vi "Startup.vi"(6 "DataQueues":refnum<class "DataQueues.lvclass">, 8 "error in (no error)":errorcluster, 10 "DAQ Settings*":T1, 11 "DAQ":refnum<class "DAQ.lvclass">) -> (0 "error out":errorcluster, 3 "DAQ":refnum<class "DAQ.lvclass">)   [LabVIEW 2022 SP3, in "DAQ.lvclass"]
doc: "Developed by Kevin Thompson\nkevin@thompsonengineering.net\n\nCopyright 2018-2020\nThompson Engineering, LLC"
uses:
  DAQ.lvclass
  Support/DataQueues/DataQueues.lvclass
  DataTypes/TD DAQ Settings--cluster.ctl
  DataTypes/TD DI Instrument Settings--cluster.ctl
  DataTypes/TD AI Instrument Settings--cluster.ctl
  DataTypes/TD AI InstSettings--cluster.ctl
  Process/ProcessSupport/TD SimAI Ranges--cluster.ctl
  DataTypes/TD DAQ&TDMS State Data--cluster.ctl
  DataTypes/TD DaqState--enum.ctl
  DataTypes/Dependency--cluster.ctl
  DAQ.lvclass/DAQ.ctl
  Accessors/Set DAQNodes Dict.vi
  Accessors/Set DAQData Dict.vi
  Accessors/Set DAQ&TDMS State Data.vi
  Accessors/Set DAQ Settings.vi
  Accessors/Set Dependency.vi
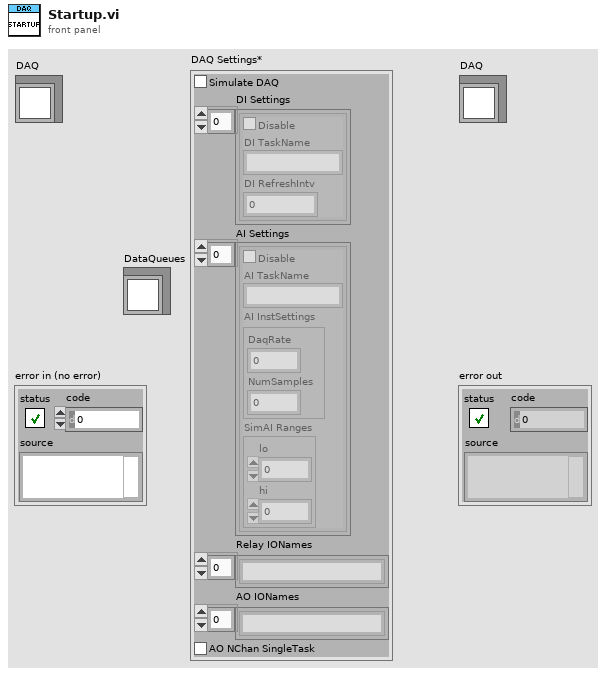
[diagram p1: front panel]
types:
  T1 = typedef "DAQ.lvclass/TD DAQ Settings--cluster.ctl" = cluster{"Simulate DAQ":bool, "DI Settings":T2[], "AI Settings":T3[], "Relay IONames":string[], "AO IONames":string[], "AO NChan SingleTask":bool}
  T2 = typedef "DAQ.lvclass/TD DI Instrument Settings--cluster.ctl" = cluster{"Disable":bool, "DI TaskName":string, "DI RefreshIntv":i32}
  T3 = typedef "DAQ.lvclass/TD AI Instrument Settings--cluster.ctl" = cluster{"Disable":bool, "AI TaskName":string, "AI InstSettings":T4, "SimAI Ranges":T5}
  T4 = typedef "DAQ.lvclass/TD AI InstSettings--cluster.ctl" = cluster{"DaqRate":dbl, "NumSamples":i32}
  T5 = typedef "DAQ.lvclass/TD SimAI Ranges--cluster.ctl" = cluster{"lo":dbl, "hi":dbl}
  T6 = typedef "DAQ.lvclass/Dependency--cluster.ctl" = cluster{"DataQueues":refnum<class "DataQueues.lvclass">}
  T7 = typedef "DAQ.lvclass/TD DAQ&TDMS State Data--cluster.ctl" = cluster{"DAQState":T8, "vData":variant}
  T8 = typedef "DAQ.lvclass/TD DaqState--enum.ctl" = enum16{"Unknown", "Stopped", "Running", "Error"}
  T9 = typedef "TD Dynamic CVT DVR--ref.ctl" = refnum<data-value>
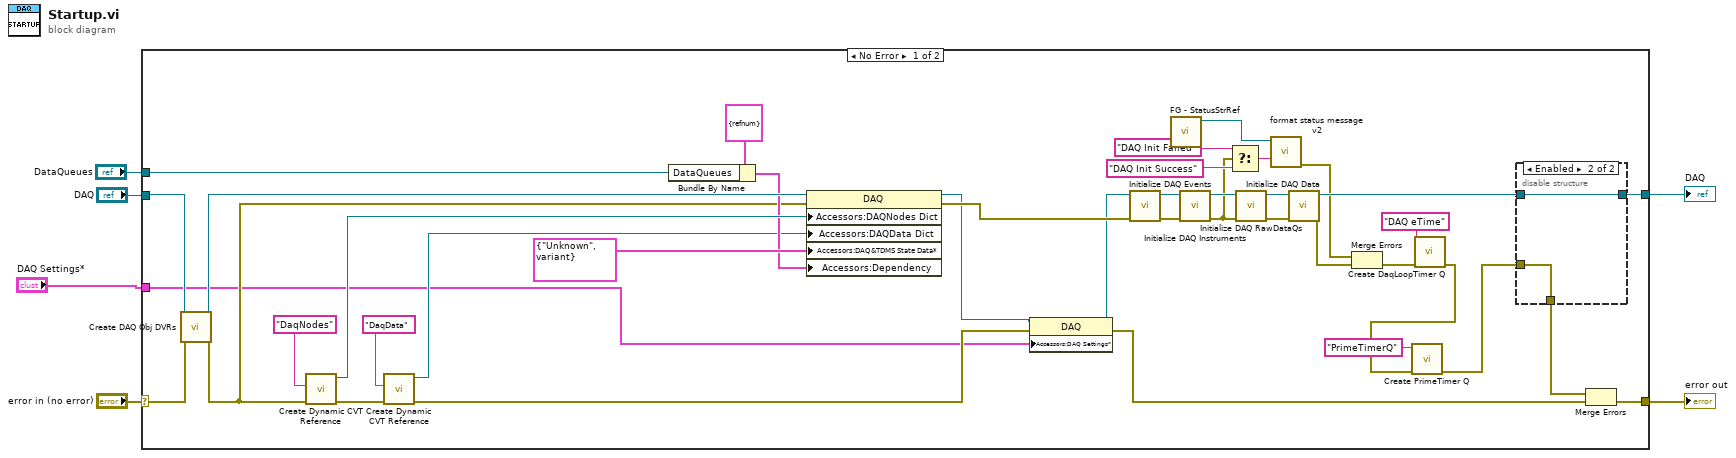
[diagram p0: block diagram]
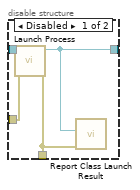
[diagram p2: hidden frame]
diagram:
  n1 = case shown="No Error" "error in (no error)" {
    selector: "error in (no error)" -> [w37 w54]
    tunnel: [w40 w54] -> w5
    tunnel: [w22 w53] -> w3
    tunnel: "DAQ" -> [w36 w53]
    tunnel: "DataQueues" -> [w24 _]
    tunnel: "DAQ Settings*" -> [w10 _]
    frame No Error {
      n2 = call "Create DAQ Obj DVRs.vi"("error in (no error)"=w37, "DAQ in"=w36) -> ("error out"=w13:errorcluster, "DAQ out"=w35:refnum<class "DAQ.lvclass">)  [unwired: 8 in]
      n3 = call <vilib>:"Create Dynamic CVT Reference.vi"("error in (no error)"=w13, "DictName"="DaqNodes") -> ("error out"=w44:errorcluster, "dCVT DVR out"=w27:T9)  [unwired: 8 in]
      n4 = call <vilib>:"Create Dynamic CVT Reference.vi"("error in (no error)"=w44, "DictName"="DaqData") -> ("error out"=w11:errorcluster, "dCVT DVR out"=w14:T9)  [unwired: 8 in]
      n5 = Bundle By Name(cluster=T6 {"DataQueues"=refnum} ("Dependency"), "DataQueues"=w24) -> (w25:T6)
      n6 = property class="DAQ"(reference=w35, error in=w13, "Accessors:DAQNodes Dict"=w27, "Accessors:DAQData Dict"=w14, "Accessors:DAQ&TDMS State Data*"=T7 {"DAQState"=enum."Unknown", "vData"=variant} ("DAQ&TDMS State Data"), "Accessors:Dependency"=w25) -> (reference out=w12:refnum<class "DAQ.lvclass">, error out=w39:errorcluster)
      n7 = property class="DAQ"(reference=w12, error in=w11, "Accessors:DAQ Settings*"=w10) -> (reference out=w34:refnum<class "DAQ.lvclass">, error out=w33:errorcluster)
      n8 = call "Initialize DAQ Events.vi"("error in (no error)"=w39, "DAQ"=w34) -> ("error out"=w29:errorcluster, "DAQ"=w30:refnum<class "DAQ.lvclass">)  [unwired: 8 in]
      n9 = call "FG - StatusStrRef.vi"() -> ("StatusStr Ref out"=w21:refnum<vi>)  [unwired: 9 in, 1 out]
      n10 = call "Initialize DAQ Instruments.vi"("error in (no error)"=w29, "DAQ"=w30) -> ("error out"=w18:errorcluster, "DAQ"=w31:refnum<class "DAQ.lvclass">)  [unwired: 8 in]
      n11 = Select(t="DAQ Init Failed", s=w18, f="DAQ Init Success") -> (s? t:f=w17:string)
      n12 = call "Initialize DAQ RawDataQs.vi"("error in (no error)"=w18, "DAQ"=w31) -> ("error out"=w28:errorcluster, "DAQ"=w32:refnum<class "DAQ.lvclass">)  [unwired: 8 in]
      n13 = call <vilib>:"format status message v2.vi"("status msg"=w17, "Str Refnum"=w21) -> ("error out"=w15:errorcluster)  [unwired: 5 in, 4 out]
      n14 = call "Initialize DAQ Data.vi"("error in (no error)"=w28, "DAQ"=w32) -> ("error out"=w41:errorcluster, "DAQ"=w42:refnum<class "DAQ.lvclass">)  [unwired: 8 in]
      n15 = Merge Errors(w15, w41) -> (w16:errorcluster)
      n16 = call "Create DaqLoopTimer Q.vi"("error in (no error)"=w16, "QName"="DAQ eTime") -> ("error out"=w7:errorcluster)  [unwired: 8 in, 1 out]
      n17 = call "Create PrimeTimer Q.vi"("error in (no error)"=w7, "QName"="PrimeTimerQ") -> ("error out"=w8:errorcluster)  [unwired: 8 in, 1 out]
      n18 = disable-structure shown="Enabled" {
        disable-tunnel: w8 -> [w50 w51]
        disable-tunnel: w42 -> [w49 w52]
        disable-tunnel: [w48 w51] -> w23
        disable-tunnel: [w47 w52] -> w22
        frame Disabled {
          n19 = call "Launch Process.vi"("error in (no error)"=w50, "DAQ"=w49) -> ("error out"=w48:errorcluster, "DAQ"=w47:refnum<class "DAQ.lvclass">)  [unwired: 8 in]
          n20 = call "Report Class Launch Result.vi"("Object"=w47, "error in (no error)"=w48) -> ()  [unwired: 8 in, 1 out]
        }
        frame Enabled {
        }
      }
      n21 = Merge Errors(w23, w33) -> (w40:errorcluster)
    }
    frame Error {
    }
  }
  "error out" <- w5
  "DAQ" <- w3
